vi "Find subWorkers - Recursive.vi"(11 "subWorkers":refnum<class "Worker.lvclass">[](array[class])) -> (2 "WIDs":string[](array[string]), 3 "Elements in Queue":i32[](array[numeric]))   [LabVIEW 2017, in "_Check all Worker Queues.lvclass"]
doc: "Iterates through the entire Worker application to check the number of elements in each Worker Queue"
uses:
  _Check all Worker Queues.lvclass
  <vilib>/addons/_Workers/Library/Classes/Worker/Worker.lvclass
  <vilib>/addons/_Workers/Library/Classes/Message Queue/Message Queue.lvclass
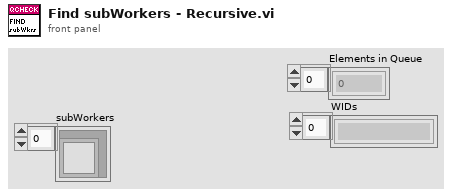
[diagram p1: front panel]
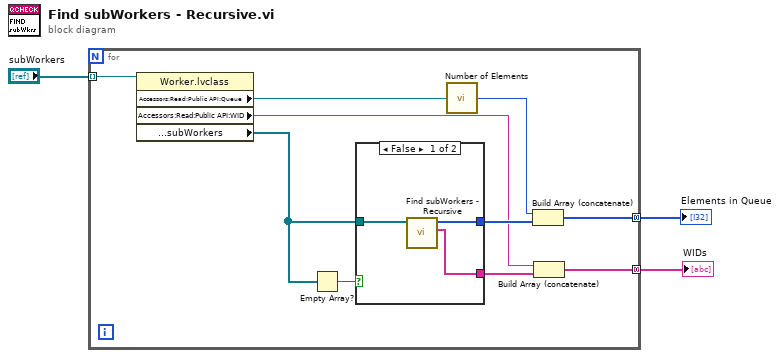
[diagram p0: block diagram]
diagram:
  n1 = for {
    tunnel: "subWorkers" -> [w12] mode=indexing
    tunnel: [w8] -> w1 mode=concatenating
    tunnel: [w5] -> w2 mode=concatenating
    n2 = property class="Worker.lvclass"(reference=w12) -> ("Accessors:Read:Public API:Queue"=w13:refnum<class "Message Queue.lvclass">, "Accessors:Read:Public API:WID"=w6:string, "Accessors:Read:Public API:subWorkers"=w10:refnum<class "Worker.lvclass">[])  [unwired: 1 in, 2 out]
    n3 = Empty Array?(array=w10) -> (empty?=w11:bool)
    n4 = case shown="False" w11 {
      tunnel: w10 -> [w16 _]
      tunnel: [w15 _] -> w9
      tunnel: [w14 _] -> w7
      frame False {
        n5 = call "Find subWorkers - Recursive.vi"("subWorkers"=w16) -> ("WIDs"=w14:string[], "Elements in Queue"=w15:i32[])  [unwired: 9 in]
      }
      frame True {
      }
    }
    n6 = call <vilib>:"Number of Elements.vi"("Message Queue"=w13) -> ("Elements in Queue"=w4:i32)  [unwired: 8 in]
    n7 = Build Array (concatenate)(w4, w9) -> (w8:i32[])
    n8 = Build Array (concatenate)(w6, w7) -> (w5:string[])
  }
  "Elements in Queue" <- w1
  "WIDs" <- w2
